vi "GUICalibrationManager_Init.vi"(8 "error in (no error)":errorcluster, 11 "GUI_About in":refnum<class "CalibrationManagerActor.lvclass">) -> (0 "error out":errorcluster, 3 "GUI_About out":refnum<class "CalibrationManagerActor.lvclass">)   [LabVIEW 2017, in "CalibrationManagerActor.lvlib" / "CalibrationManagerActor.lvclass"]
uses:
  CalibrationManagerActor.lvclass
  CalibrationManagerActor.lvclass/CalibrationManagerActor.ctl
  Library/Amfax Library/Amfax Library/AmFax Source Code.lvclass
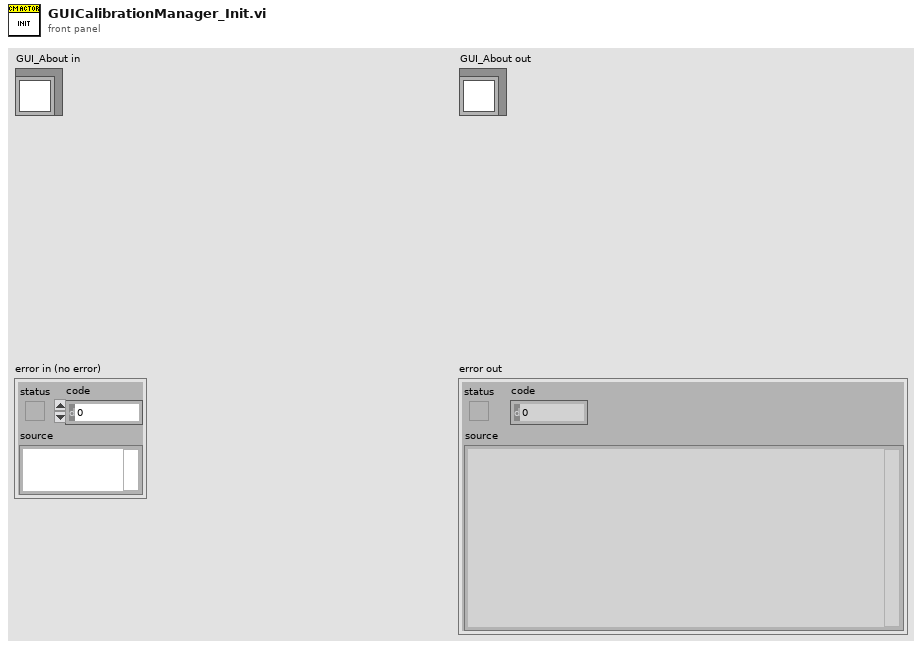
[diagram p1: front panel]
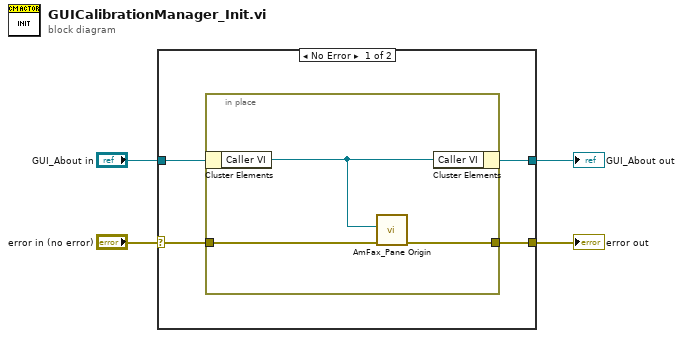
[diagram p0: block diagram]
diagram:
  n1 = case shown="No Error" "error in (no error)" {
    selector: "error in (no error)" -> [w8 w13]
    tunnel: [w7 w13] -> w3
    tunnel: [w5 w12] -> w1
    tunnel: "GUI_About in" -> [w6 w12]
    frame No Error {
      n2 = in-place {
        in-place-border: w8 -> [w10]
        in-place-border: [w9] -> w7
        n3 = in-place-cluster #1(w6) -> ("Caller VI"=w11:refnum<vi>)
        n4 = call "AmFax_Pane Origin.vi"("error in (no error)"=w10, "This VI"=w11) -> ("error out"=w9:errorcluster)  [unwired: 8 in, 1 out]
        n5 = in-place-cluster #1("Caller VI"=w11) -> (w5:refnum<class "CalibrationManagerActor.lvclass">)
      }
    }
    frame Error {
    }
  }
  "error out" <- w3
  "GUI_About out" <- w1
